vi "UI.vi"(0 "Subtract in":refnum<class "Subtract.lvclass">, 5 "Num 1":dbl, 7 "Num 2":dbl, 11 "Error In":errorcluster) -> (4 "Subtract out":refnum<class "Subtract.lvclass">, 6 "Output":dbl, 15 "Error Out":errorcluster)   [LabVIEW 2020, in "Subtract.lvclass"]
doc: "This method will handle the UI Operations."
uses:
  Subtract.lvclass
  D:/Github Projects/LV_Assignment/Tasks/A18/A18/Classes/Arithmetic_Operations/Arithmetic_Operations.lvclass
  Typedef's/UserEvent_Operations.ctl
  Subtract.lvclass/Subtract.ctl
  Arithmetic_Operations/Arithmetic_Operations.lvclass
  Calculator_Using_Objects.lvlib
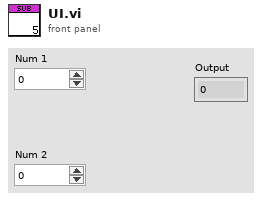
[diagram p1: front panel]
types:
  T1 = typedef "Calculator_Using_Objects.lvlib/UserEvent_Operations.ctl" = enum16{"Create", "Generate", "Get Ref", "Destroy"}
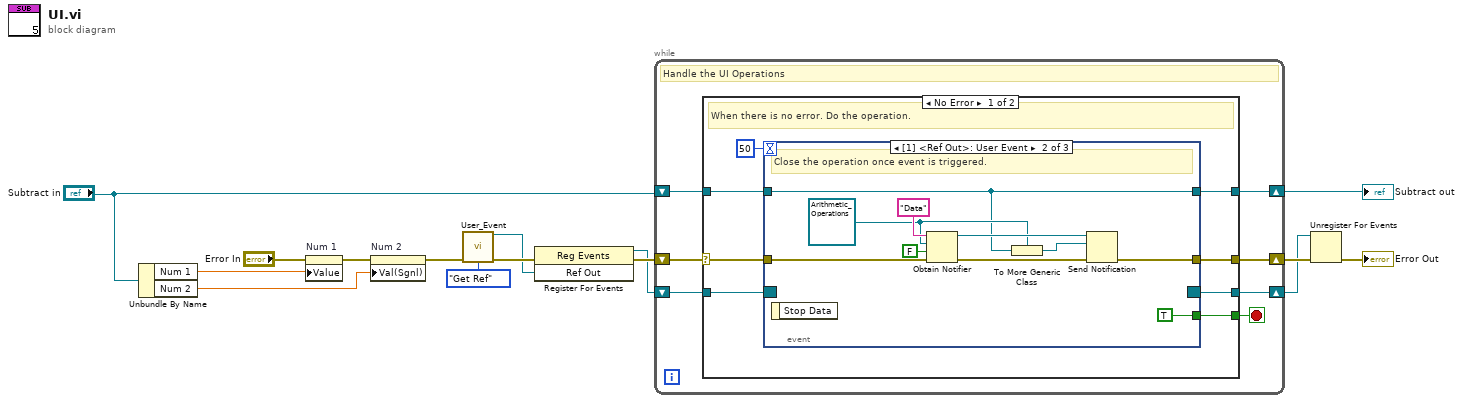
[diagram p0: block diagram]
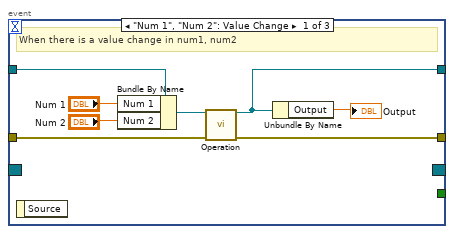
[diagram p2: hidden frame]
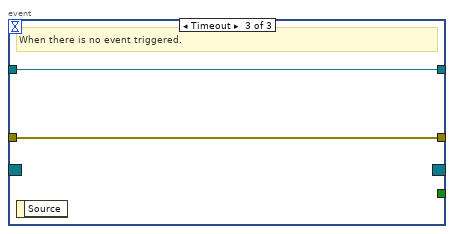
[diagram p3: hidden frame]
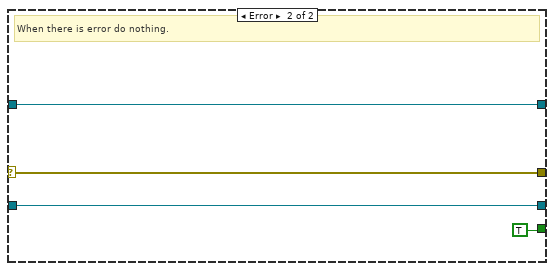
[diagram p4: hidden frame]
diagram:
  n1 = Unbundle By Name("Subtract in") -> ("Num 1"=w4:dbl, "Num 2"=w3:dbl)
  n2 = property on="Num 1" class="DigNum (strict)"(error in="Error In", "Value"=w4) -> (error out=w5:errorcluster)  [unwired: 1 in, 1 out]
  n3 = property on="Num 2" class="DigNum (strict)"(error in=w5, "Val(Sgnl)"=w3) -> (error out=w13:errorcluster)  [unwired: 1 in, 1 out]
  n4 = call "User_Event.vi"("Error In"=w13, "Enum"=UserEvent_Operations."Get Ref") -> ("Ref Out"=w9:refnum<user-event>, "Error Out"=w12:errorcluster)  [unwired: 12 in]
  n5 = register-events(error in=w12, w9) -> (reference out=w8:refnum<event-registration>, error out=w10:errorcluster)  [unwired: 1 in]
  n6 = while {
    shift-right: [w20] -> w14
    shift-left: w10 -> [w22]
    shift-right: [w19] -> w1
    shift-left: "Subtract in" -> [w21]
    shift-right: [w17] -> w6
    shift-left: w8 -> [w18]
    stop <- w16 stop-if-true
    # "Handle the UI Operations"
    n7 = case shown="No Error" w22 {
      selector: w22 -> [w30 w53]
      tunnel: w21 -> [w29 w54]
      tunnel: [w28 w53] -> w20
      tunnel: [w27 w54] -> w19
      tunnel: w18 -> [w25 w52]
      tunnel: [w24 w52] -> w17
      tunnel: [w23 TRUE] -> w16
      frame No Error {
        # "When there is no error. Do the operation."
        n8 = event shown="[1] <Ref Out>: User Event" {
          selector: w25 -> [_ _ _]
          dyn-events: [_ _ _] -> w24
          timeout: 50 -> [_ _ _]
          tunnel: w30 -> [w33 w41 w49]
          tunnel: w29 -> [w38 w40 w50]
          tunnel: [w34 w42 w49] -> w28
          tunnel: [w32 w40 w50] -> w27
          tunnel: [_ TRUE _] -> w23
          event "Num 1", "Num 2": Value Change {
            # "When there is a value change in num1, num2"
            n9 = event-data() -> ()  [unwired: 1 in, 1 out]
            n10 = Bundle By Name(cluster=w38, "Num 1"="Num 1", "Num 2"="Num 2") -> (w35:refnum<class "Subtract.lvclass">)
            n11 = call-dynamic "Operation.vi"("Subtract in"=w35, "Error In"=w33) -> ("Subtract out"=w32:refnum<class "Subtract.lvclass">, "Error Out"=w34:errorcluster)  [unwired: 12 in]
            n12 = Unbundle By Name(w32) -> ("Output"=→"Output":dbl)
          }
          event User Event {
            w44 = refnum<class "Arithmetic_Operations.lvclass"> refnum ("Arithmetic_Operations.lvclass")
            # "Close the operation once event is triggered."
            n13 = event-data() -> ()  [unwired: 1 in, 1 out]
            n14 = Obtain Notifier(name (unnamed)="Data", notification data type=w44, create if not found? (T)=FALSE, error in (no error)=w41) -> (notifier out=w45:refnum<notifier>, error out=w39:errorcluster)  [unwired: 1 out]
            n15 = To More Generic Class(target class=w44, reference=w40) -> (generic class reference=w43:refnum<class "Arithmetic_Operations.lvclass">)
            n16 = Send Notification(notification=w43, notifier=w45, error in (no error)=w39) -> (error out=w42:errorcluster)  [unwired: 1 out]
          }
          event Timeout {
            # "When there is no event triggered."
            n17 = event-data() -> ()  [unwired: 1 in, 1 out]
          }
        }
      }
      frame Error {
        # "When there is error do nothing."
      }
    }
  }
  "Subtract out" <- w1
  n18 = Unregister For Events(event registration refnum=w6, error in=w14) -> (error out=→"Error Out":errorcluster)
